vi "Wrap BD in Error Case - Plugin -.vi"(8 "error in":errorcluster) -> (0 "error out":errorcluster)   [LabVIEW 2018]
uses:
  <vilib>/addons/_JKI Toolkits/RCF API/Right Click API.llb/Generic Option - Input Data - __RightClickAPI.ctl
  <vilib>/addons/_JKI Toolkits/RCF API/Right Click API.llb/Right Click API Menu Activation Data__RightClickAPI.ctl
  <vilib>/picture/picture.llb/imagedata.ctl
  <vilib>/addons/_JKI Toolkits/RCF API/Right Click API.llb/Right Click API Plugin Info Data__RightClickAPI.ctl
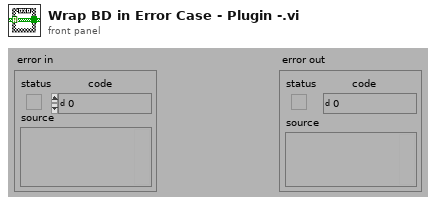
[diagram p1: front panel]
types:
  T1 = typedef "RightClickAPI.lvlib/Right Click API Plugin Info Data__RightClickAPI.ctl" = cluster{"Name":string, "Summary":string, "Description":string, "Copyright":string, "License":string, "Developer":string, "Version":string, "Plugin Glyph (32x32)":T2}
  T2 = typedef "imagedata.ctl" = cluster{"image type":i32, "image depth":i32, "image":u8[], "mask":u8[], "colors":u32[], "Rectangle":cluster{"left":i16, "top":i16, "right":i16, "bottom":i16}}
  T3 = typedef "RightClickAPI.lvlib/Right Click API Framework Data__RightClickAPI.ctl" = cluster{"Active VI Info":T4, "Mode":T6, "Shortcut Menu Selection":T7, "Plugins Options":T8}
  T4 = typedef "RightClickAPI.lvlib/Framework - Active VI Info - Cluster - __RightClickAPI.ctl" = cluster{"Active VI Refnum":refnum<vi>, "Active VI Type":T5, "Active VI Sel. List[]":refnum<vi>[], "Mouse Coords":cluster{"Horizontal":i32, "Vertical":i32}}
  T5 = typedef "RightClickAPI.lvlib/Framework - Selection Type - Enum - __RightClickAPI.ctl" = enum16{"Panel", "Diagram"}
  T6 = typedef "RightClickAPI.lvlib/Right Click API - Mode - Enum - __RightClickAPI.ctl" = enum16{"Initialize", "Menu Activation", "Menu Selection", "Edit Options"}
  T7 = typedef "RightClickAPI.lvlib/Framework - Shortcut Menu Selection Events - Cluster - __RightClickAPI.ctl" = cluster{"ItemTag":string, "ItemPath":string, "Coords":cluster{"Horizontal":i32, "Vertical":i32}}
  T8 = typedef "RightClickAPI.lvlib/Framework - Plugin Options - Cluster - __RightClickAPI.ctl" = cluster{"Config Data":string}
  T9 = typedef "RightClickAPI.lvlib/Right Click API Menu Activation Data__RightClickAPI.ctl" = cluster{"Menu String":string}
  T10 = typedef "RightClickAPI.lvlib/Generic Option - Input Data - __RightClickAPI.ctl" = cluster{"Config Data":variant}
  T11 = typedef "RightClickAPI.lvlib/Generic Option - Output Data - __RightClickAPI.ctl" = cluster{"Config Data":variant}
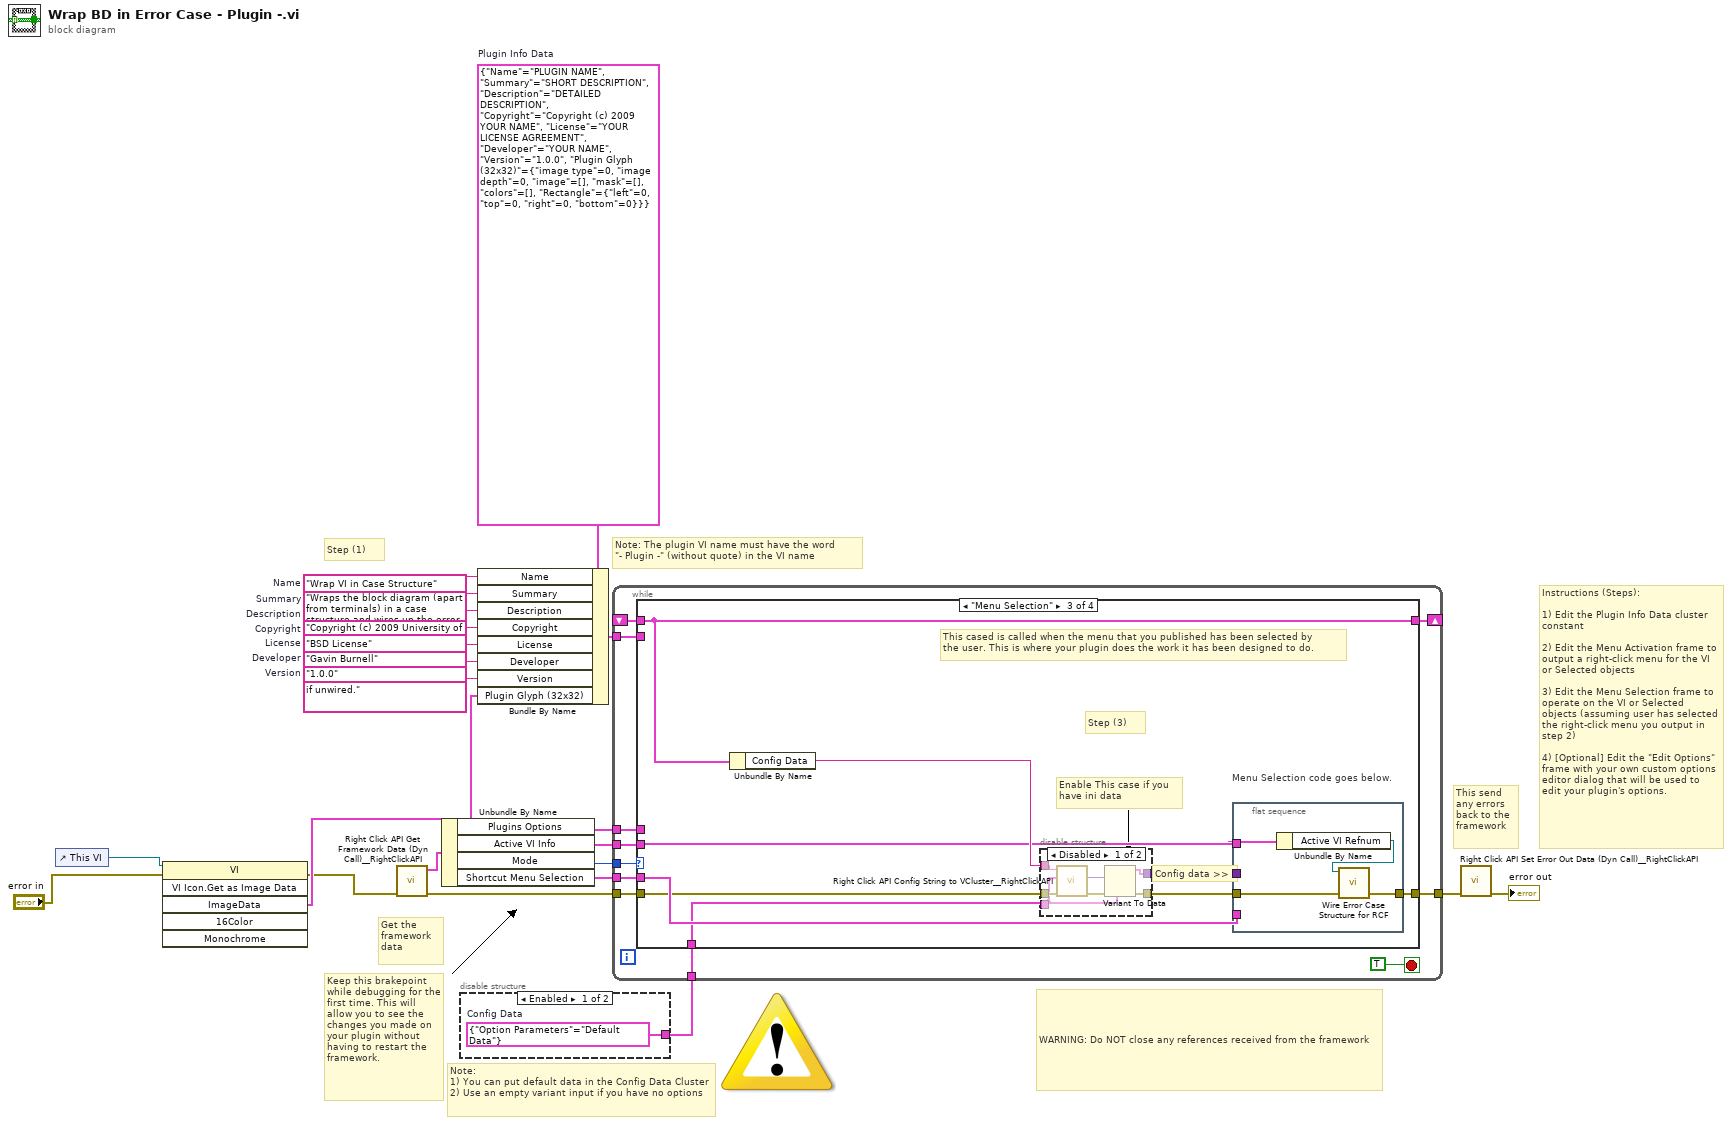
[diagram p0: block diagram]
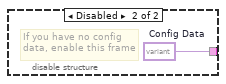
[diagram p2: hidden frame]
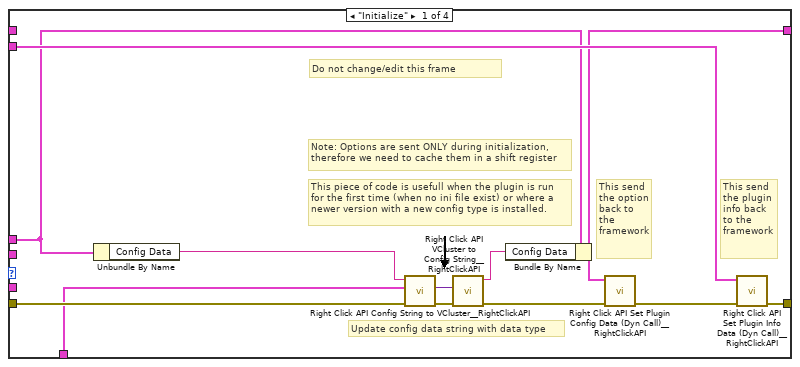
[diagram p3: hidden frame]
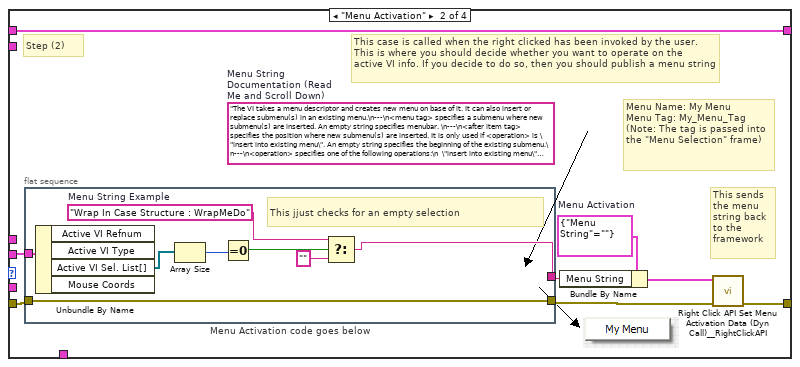
[diagram p4: hidden frame]
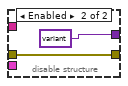
[diagram p5: hidden frame]
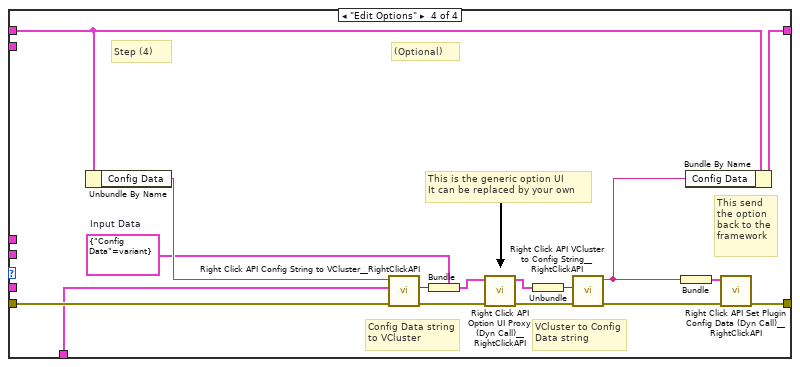
[diagram p6: hidden frame]
diagram:
  w5 = "1.0.0"  # Version
  w6 = "Gavin Burnell"  # Developer
  w7 = "BSD License"  # License
  w8 = "Copyright (c) 2009 University of Leeds, UK"  # Copyright
  w9 = "Encloses all the contents of the VI apart from control and indicator terminals ina  case structure and then looks to see if it can wire up the error wire. Sets all the other output terminals to use default values if unwired."  # Description
  w10 = "Wraps the block diagram (apart from terminals) in a case structure and wires up the error cluster."  # Summary
  w11 = "Wrap VI in Case Structure"  # Name
  w12 = T1 {"Name"="PLUGIN NAME", "Summary"="SHORT DESCRIPTION", "Description"="DETAILED DESCRIPTION", "Copyright"="Copyright (c) 2009 YOUR NAME", "License"="YOUR LICENSE AGREEMENT", "Developer"="YOUR NAME", "Version"="1.0.0", "Plugin Glyph (32x32)"={"image type"=0, "image depth"=0, "image"=[], "mask"=[], "colors"=[], "Rectangle"={"left"=0, "top"=0, "right"=0, "bottom"=0}}}  # Plugin Info Data
  # "Keep this brakepoint while debugging for the first time. This will allow you to see the changes you made on your plugin without having to restart the framework."
  # "WARNING: Do NOT close any references received from the framework"
  # "Step (1)"
  # "Instructions (Steps):\n\n1) Edit the Plugin Info Data cluster constant\n\n2) Edit the Menu Activation frame to output a right-click menu for the VI or Selected objects\n\n3) Edit the Menu Selection frame to operate on the VI or Selected objects (assuming user has selected the right-click menu you output in step 2)\n\n4) [Optional] Edit the \"Edit Options\" frame with your own custom options editor dialog that will be used to edit your plugin's options."
  # "Note: The plugin VI name must have the word \n\"- Plugin -\" (without quote) in the VI name"
  # "Get the framework data"
  # "This send any errors back to the framework"
  # "Note:\n1) You can put default data in the Config Data Cluster\n2) Use an empty variant input if you have no options"
  n1 = control-ref of="This VI"() -> (w4:refnum<vi>)
  n2 = invoke class="VI" method="VI Icon.Get as Image Data"(reference=w4, error in="error in") -> (error out=w1:errorcluster, "ImageData"=w3:T2)  [unwired: 4 in, 4 out]
  n3 = call <vilib>:"Right Click API Get Framework Data (Dyn Call)__RightClickAPI.vi"("error in (no error)"=w1) -> ("error out"=w17:errorcluster, "Framework Data"=w16:T3)  [unwired: 9 out]
  n4 = Unbundle By Name(w16) -> ("Plugins Options"=w15:T8, "Active VI Info"=w21:T4, "Mode"=w22:T6, "Shortcut Menu Selection"=w20:T7)
  n5 = disable-structure shown="Enabled" {
    disable-tunnel: [w23 w24] -> w14
    frame Enabled {
      w23 = cluster{"Option Parameters":string} {"Option Parameters"="Default Data"}  # Config Data
    }
    frame Disabled {
      w24 = variant  # Config Data
      # "If you have no config data, enable this frame"
    }
  }
  n6 = Bundle By Name(cluster=w12, "Name"=w11, "Summary"=w10, "Description"=w9, "Copyright"=w8, "License"=w7, "Developer"=w6, "Version"=w5, "Plugin Glyph (32x32)"=w3) -> (w13:T1)
  n7 = while {
    tunnel: w22 -> [w35]
    tunnel: w21 -> [w34]
    tunnel: w20 -> [w33]
    tunnel: [w32] -> w19
    tunnel: w17 -> [w31]
    tunnel: w13 -> [w30]
    shift-right: [w27] -> _
    shift-left: _ -> [w26]
    tunnel: w15 -> [w28]
    tunnel: w14 -> [w25]
    stop <- TRUE stop-if-true
    n8 = case shown="\"Menu Selection\"" w35 {
      tunnel: w31 -> [w44 w54 w69 w99]
      tunnel: [w47 w55 w72 w93] -> w32
      tunnel: w34 -> [_ w48 w64 _]
      tunnel: w33 -> [_ _ w71 _]
      tunnel: w30 -> [w46 _ _ _]
      tunnel: w28 -> [w39 _ _ _]
      tunnel: [w36 w50 w68 w100] -> w27
      tunnel: w26 -> [_ w50 w68 w101]
      tunnel: w25 -> [w42 _ w66 w98]
      frame "Initialize" {
        # "Do not change/edit this frame"
        # "Update config data string with data type"
        # "This send the plugin info back to the framework"
        # "This send the option back to the framework"
        # "This piece of code is usefull when the plugin is run for the first time (when no ini file exist) or where a newer version with a new config type is installed."
        # "Note: Options are sent ONLY during initialization, therefore we need to cache them in a shift register"
        n9 = Unbundle By Name(w39) -> ("Config Data"=w41:string)
        n10 = call <vilib>:"Right Click API Config String to VCluster__RightClickAPI.vi"("error in (no error)"=w44, "type"=w42, "Config String"=w41) -> ("error out"=w45:errorcluster, "VCluster"=w43:variant)  [unwired: 7 out]
        n11 = call <vilib>:"Right Click API VCluster to Config String__RightClickAPI.vi"("error in (no error)"=w45, "VCluster"=w43) -> ("error out"=w37:errorcluster, "Config String"=w40:string)  [unwired: 8 out]
        n12 = Bundle By Name(cluster=w39, "Config Data"=w40) -> (w36:T8)
        n13 = call <vilib>:"Right Click API Set Plugin Config Data (Dyn Call)__RightClickAPI.vi"("error in (no error)"=w37, "Plugins Options"=w36) -> ("error out"=w38:errorcluster)  [unwired: 9 out]
        n14 = call <vilib>:"Right Click API Set Plugin Info Data (Dyn Call)__RightClickAPI.vi"("error in (no error)"=w38, "Plugin Info Data"=w46) -> ("error out"=w47:errorcluster)  [unwired: 9 out]
      }
      frame "Menu Activation" {
        w49 = T9 {"Menu String"=""}  # Menu Activation
        (unwired) "The VI takes a menu descriptor and creates new menu on base of it. It can also insert or replace submenu(s) in an existing menu.\n---\n<menu tag> specifies a submenu where new submenu(s) are inserted. An empty string specifies menubar. \n---\n<after item tag> specifies the position where new submenu(s) are inserted. It is only used if <operation> is \"insert into existing menu\". An empty string specifies the beginning of the existing submenu.\n---\n<operation> specifies one of the following operations:\n  \"insert into existing menu\" inserts the new submenu(s) to <menu tag> submenu at <after item tag> position.\n  \"append to existing submenu\" appends the new submenu(s) to the end of <menu tag> submenu.\n  \"replace existing menu\" replaces all the items in the <menu tag> submenu with the new submenu(s).\n---\n<menu descriptor> is a multi-line string where each line contains a menu item attributes. Empty lines and lines beginning with semicolon (;) are ignored. A line starting with a dash sign (-) forms a separator in menu. A descriptor line has the following format:\n\n  [SubMenuSign] ItemName : ItemTag [ : ItemParams [ : comments] ]\n\nSybMenuSign is optional parameter that can be either greater-than sign (>) marking the beginning of new submenu or less-than sign (<) marking the end of submenu. If a line begins with less-than sign (<), the rest of the line is ignored. You can form nested submenus providing that each '>' block is terminated with '<'.\n\nItemNames and ItenTags are respectively a name of menu item and a tag of menu item. If an item name includes a underscore sign (_), the following character is used for ALT navigation. \n\nItemParams can contain optional specificators of the menu item separated by spaces. The specificators are not case-sensitive. You can use the following specificators:\nDIS - menu item is disabled\nCHK - menu item is checked\nKEY=CHAR - specifies a shortcut keys combination. If CHAR begins with '@' sign, the shortcut is CTRL-SHIFT-CHAR; otherwise, it is CTRL-CHAR.\n\nExample:\n------------\n; File menu\n> File : file\n  _Open... : open : key=O\n  _Close... : close : key=C\n  -  ;separator\n  ; nested submenu\n  > Configuration : config\n    Parameter 1 : cfg_1 : CHK : checked\n    Parameter 2 : cfg_2 : DIS : disabled\n  <\n  -  ;separator\n  E_xit : exit : key=X\n<\n; Mode menu\n> Mode : mode\nmode 1 : mode1 : KEY=@A CHK\nmode 2 : mode2 : KEY=@B DIS\nmode 3 : mode3 : KEY=@C\n<\n"  # Menu String Documentation (Read Me and Scroll Down)
        # "Menu Name: My Menu\nMenu Tag: My_Menu_Tag\n(Note: The tag is passed into the \"Menu Selection\" frame)"
        # "Step (2)"
        # "This sends the menu string back to the framework"
        # "This case is called when the right clicked has been invoked by the user.\nThis is where you should decide whether you want to operate on the \nactive VI info. If you decide to do so, then you should publish a menu string"
        n15 = flat-sequence "Menu Activation code goes below" {
          tunnel: w54 -> [w63]
          tunnel: [w63] -> w53
          tunnel: [w57] -> w52
          tunnel: w48 -> [w62]
          frame #0 {
            w58 = "Wrap In Case Structure : WrapMeDo"  # Menu String Example
            # "This jjust checks for an empty selection"
            n16 = Unbundle By Name(w62) -> ("Active VI Sel. List[]"=w61:refnum<vi>[])  [unwired: 3 out]
            n17 = Array Size(array=w61) -> (size(s)=w60:i32)
            n18 = Equal To 0?(x=w60) -> (x = 0?=w59:bool)
            n19 = Select(t=w58, s=w59, f="") -> (s? t:f=w57:string)
          }
        }
        n20 = Bundle By Name(cluster=w49, "Menu String"=w52) -> (w51:T9)
        n21 = call <vilib>:"Right Click API Set Menu Activation Data (Dyn Call)__RightClickAPI.vi"("error in (no error)"=w53, "Menu Activation Data"=w51) -> ("error out"=w55:errorcluster)  [unwired: 9 out]
      }
      frame "Menu Selection" {
        # "Step (3)"
        # "Enable This case if you \nhave ini data"
        # "Config data >>"
        # "This cased is called when the menu that you published has been selected by\nthe user. This is where your plugin does the work it has been designed to do."
        n22 = Unbundle By Name(w68) -> ("Config Data"=w67:string)
        n23 = disable-structure shown="Disabled" {
          disable-tunnel: [w77 w81] -> w70
          disable-tunnel: w69 -> [w76 w81]
          disable-tunnel: w67 -> [w75 _]
          disable-tunnel: w66 -> [w74 _]
          disable-tunnel: [w73 variant ("Config Type")] -> w65
          frame Disabled {
            n24 = call <vilib>:"Right Click API Config String to VCluster__RightClickAPI.vi"("error in (no error)"=w76, "type"=w74, "Config String"=w75) -> ("error out"=w79:errorcluster, "VCluster"=w78:variant)  [unwired: 7 in]
            n25 = Variant To Data(error in=w79, type=w74, Variant=w78) -> (data=w73:cluster{"Option Parameters":string}, error out=w77:errorcluster)
          }
          frame Enabled {
          }
        }
        n26 = flat-sequence "Menu Selection code goes below." {
          tunnel: w64 -> [w83]
          tunnel: w70 -> [w85]
          tunnel: [w84] -> w72
          tunnel: w71 -> [_]
          tunnel: w65 -> [_]
          frame #0 {
            n27 = Unbundle By Name(w83) -> ("Active VI Refnum"=w82:refnum<vi>)
            n28 = call "Wire Error Case Structure for RCF.vi"("error in (no error)"=w85, "Vi Ref"=w82) -> ("error out"=w84:errorcluster)  [unwired: 9 out]
          }
        }
      }
      frame "Edit Options" {
        w90 = T10 {"Config Data"=variant}  # Input Data
        # "Step (4)"
        # "(Optional)"
        # "VCluster to Config Data string"
        # "Config Data string to VCluster"
        # "This send the option back to the framework"
        # "This is the generic option UI\nIt can be replaced by your own"
        n29 = Unbundle By Name(w101) -> ("Config Data"=w97:string)
        n30 = call <vilib>:"Right Click API Config String to VCluster__RightClickAPI.vi"("error in (no error)"=w99, "type"=w98, "Config String"=w97) -> ("error out"=w96:errorcluster, "VCluster"=w89:variant)  [unwired: 7 out]
        n31 = Bundle(cluster=w90, "Config Data"=w89) -> (w88:T10)
        n32 = call <vilib>:"Right Click API Option UI Proxy (Dyn Call)__RightClickAPI.vi"("error in (no error)"=w96, "Input Data"=w88) -> ("error out"=w95:errorcluster, "Output Data"=w87:T11)  [unwired: 8 out]
        n33 = Unbundle(w87) -> ("Config Data"=w86:variant)
        n34 = call <vilib>:"Right Click API VCluster to Config String__RightClickAPI.vi"("error in (no error)"=w95, "VCluster"=w86) -> ("error out"=w94:errorcluster, "Config String"=w92:string)  [unwired: 8 out]
        n35 = Bundle("Config String"=w92) -> (w91:cluster{"Config String":string})  [unwired: 1 in]
        n36 = Bundle By Name(cluster=w101, "Config Data"=w92) -> (w100:T8)
        n37 = call <vilib>:"Right Click API Set Plugin Config Data (Dyn Call)__RightClickAPI.vi"("error in (no error)"=w94, "Plugins Options"=w91) -> ("error out"=w93:errorcluster)  [unwired: 9 out]
      }
    }
  }
  n38 = call <vilib>:"Right Click API Set Error Out Data (Dyn Call)__RightClickAPI.vi"("error in (no error)"=w19) -> ("error out"=→"error out":errorcluster)  [unwired: 10 out]
